vi "Rotation Matrix to Quaternion.vi"(8 "error in (no error)":errorcluster, 11 "Rotation Matrix":T1) -> (0 "error out":errorcluster, 3 "Quaternion":T2)   [LabVIEW 2020, in "ar.lvlib"]
doc: "Convert a 3x3 Rotation Matrix to a normalized Quaternion."
uses:
  ar.lvlib
  Quaternion.ctl
  <vilib>/Analysis/Matrix/Datatypes/RealMatrix.ctl
  common/common.lvlib
  common/bin/gartoolkit_ar_32-1.dll
  <vilib>/Analysis/Matrix/NI_Matrix.lvlib
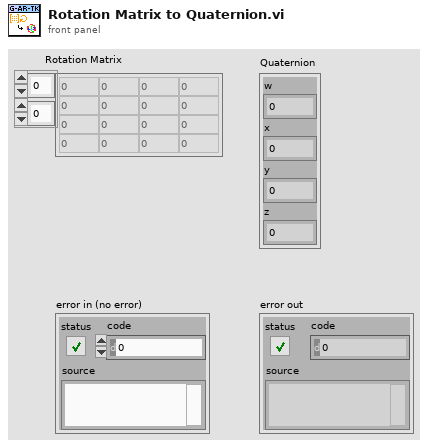
[diagram p1: front panel]
types:
  T1 = typedef "NI_Matrix.lvlib/RealMatrix.ctl" = dbl[][]
  T2 = typedef "ar.lvlib/Quaternion.ctl" = cluster{"w":dbl, "x":dbl, "y":dbl, "z":dbl}
  T3 = cluster{"Rotation Matrix[0]":dbl, "Rotation Matrix[1]":dbl, "Rotation Matrix[2]":dbl, "Rotation Matrix[3]":dbl, "Rotation Matrix[4]":dbl, "Rotation Matrix[5]":dbl, "Rotation Matrix[6]":dbl, "Rotation Matrix[7]":dbl, "Rotation Matrix[8]":dbl}
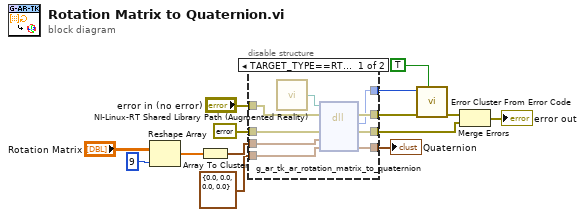
[diagram p0: block diagram]
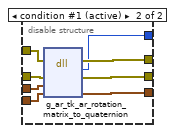
[diagram p2: hidden frame]
diagram:
  n1 = Reshape Array("Rotation Matrix", 9 ("dimension size")) -> (w11:dbl[])
  n2 = Array To Cluster(array=w11) -> (cluster=w7:T3)
  n3 = disable-structure shown="TARGET_TYPE==RT&&OS==Linux" {
    disable-tunnel: "error in (no error)" -> [w23 w31]
    disable-tunnel: errorcluster {"status"=FALSE, "code"=0, "source"=""} ("error constant") -> [w22 w30]
    disable-tunnel: w7 -> [w21 w29]
    disable-tunnel: T2 {"w"=0.0, "x"=0.0, "y"=0.0, "z"=0.0} ("Quaternion") -> [w20 w28]
    disable-tunnel: [w19 w27] -> w5
    disable-tunnel: [w18 w26] -> w4
    disable-tunnel: [w17 w25] -> w3
    disable-tunnel: [w16 w24] -> w2
    frame condition #0 {
      n4 = call "NI-Linux-RT Shared Library Path (Augmented Reality).vi"() -> ("Path"=w15:path)
      n5 = dll-call lib="?" fn="g_ar_tk_ar_rotation_matrix_to_quaternion" ("g_ar_toolkit.*.*:g_ar_tk_image_copy")(path in=w15, error in=w23, "error_cluster"=w22, "rmat"=w21, "quaternion"=w20) -> (error out=w19:errorcluster, w18:i32, "error_cluster"=w17:errorcluster, "quaternion"=w16:T2)  [unwired: 2 in, 1 out]
    }
    frame condition #1 (active) {
      n6 = dll-call lib="C:/serenial/lib/g-augmented-reality-toolkit/LabVIEW/common/bin/gartoolkit_ar_*-1.*" fn="g_ar_tk_ar_rotation_matrix_to_quaternion" ("g_ar_toolkit.*.*:g_ar_tk_image_copy")(error in=w31, "error_cluster"=w30, "rmat"=w29, "quaternion"=w28) -> (error out=w27:errorcluster, w26:i32, "error_cluster"=w25:errorcluster, "quaternion"=w24:T2)  [unwired: 3 in, 1 out]
    }
  }
  "Quaternion" <- w2
  n7 = call <vilib>:"Error Cluster From Error Code.vi"("show call chain? (False)"=TRUE, "error in (no error)"=w5, "error code (0)"=w4) -> ("error out"=w14:errorcluster)  [unwired: 6 in]
  n8 = Merge Errors(w14, w3) -> (→"error out":errorcluster)
